vi "Local Error Handler.vi"(8 "error in":errorcluster, 11 "Stop in":bool) -> (0 "error out":errorcluster, 3 "Stop out":bool)   [LabVIEW 2014, in "Daqmx Module editor node.lvclass"]
doc: "Any errors should be handled in this VI. The default behavior is to clear all errors."
uses:
  Daqmx Module editor node.lvclass
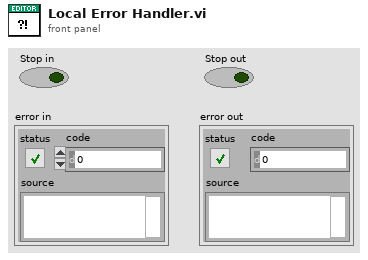
[diagram p1: front panel]
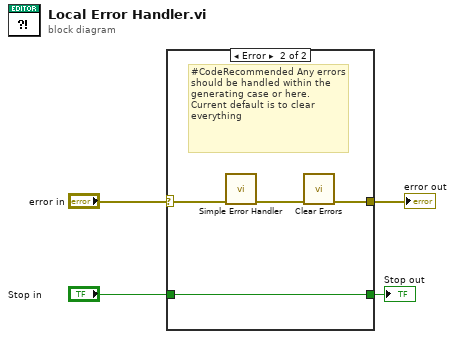
[diagram p0: block diagram]
diagram:
  n1 = case shown="Error" "error in" {
    selector: "error in" -> [w5 w9]
    tunnel: [w6 w10] -> w1
    tunnel: "Stop in" -> [w6 w10]
    tunnel: [w5 w7] -> w3
    frame No Error {
    }
    frame Error {
      # "#CodeRecommended Any errors should be handled within the generating case or here. Current default is to clear everything"
      n2 = call <vilib>:"Simple Error Handler.vi"("error in (no error)"=w9) -> ("error out"=w8:errorcluster)  [unwired: 4 in, 4 out]
      n3 = call <vilib>:"Clear Errors.vi"("error in (no error)"=w8) -> ("error out"=w7:errorcluster)  [unwired: 5 in, 1 out]
    }
  }
  "error out" <- w3
  "Stop out" <- w1
